vi "Send UUTSupply Event.vi"(8 "error in":errorcluster, 9 "Output":bool, 10 "Supply":string, 11 "Engine in":refnum<class "Engine.lvclass">) -> (0 "error out":errorcluster, 3 "Engine out":refnum<class "Engine.lvclass">)   [LabVIEW 2019, in "Engine.lvlib" / "Engine.lvclass"]
doc: "Generate an event consumed by the Chronometer to track devices that are powered on or off."
uses:
  Project/Engine.lvclass
  Project/Engine.lvclass/Engine.ctl
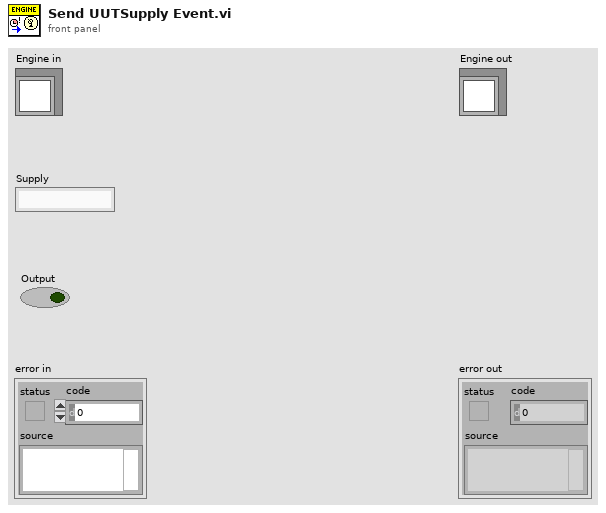
[diagram p1: front panel]
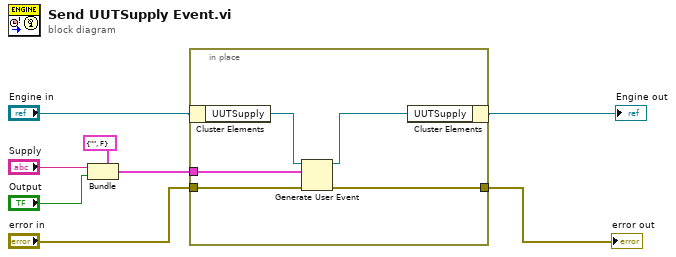
[diagram p0: block diagram]
diagram:
  n1 = Bundle(cluster=cluster{"Supply":string, "Output":bool} {"Supply"="", "Output"=FALSE} ("event data"), "Supply"="Supply", "Output"="Output") -> (w7:cluster{"Supply":string, "Output":bool})
  n2 = in-place {
    in-place-border: w7 -> [w13]
    in-place-border: "error in" -> [w10]
    in-place-border: [w9] -> w1
    n3 = in-place-cluster #1("Engine in") -> ("UUTSupply"=w12:refnum<user-event>)
    n4 = Generate User Event(user event=w12, event data cluster=w13, error in=w10) -> (user event out=w11:refnum<user-event>, error out=w9:errorcluster)  [unwired: 1 in]
    n5 = in-place-cluster #1("UUTSupply"=w11) -> (→"Engine out":refnum<class "Engine.lvclass">)
  }
  "error out" <- w1
